vi "ConnectReseauDataManager.vi"(2 "entrée d'erreur":errorcluster) -> (0 "sortie d'erreur":errorcluster, 1 "Existe?":bool)   [LabVIEW 2017]
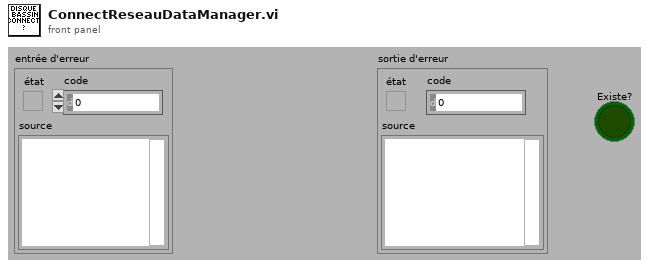
[diagram p1: front panel]
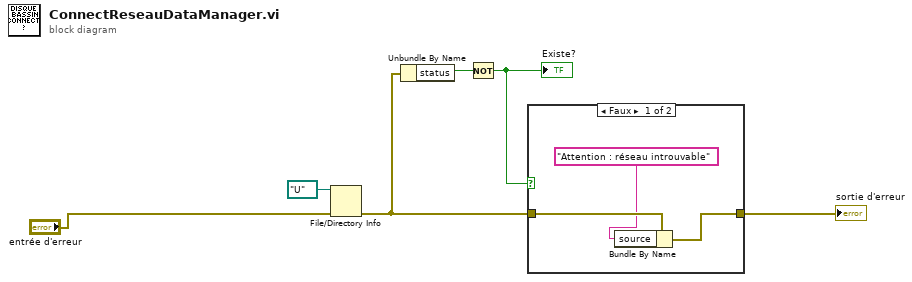
[diagram p0: block diagram]
diagram:
  n1 = File/Directory Info(path=path "U:/" ("chemin"), error in="entrée d'erreur") -> (error out=w4:errorcluster)  [unwired: 6 out]
  n2 = Unbundle By Name(w4) -> ("status"=w5:bool)
  n3 = Not(x=w5) -> (.not. x?=w6:bool)
  "Existe?" <- w6
  n4 = case shown="Faux" w6 {
    tunnel: w4 -> [w9 w10]
    tunnel: [w7 w10] -> w3
    frame False {
      n5 = Bundle By Name(cluster=w9, "source"="Attention : réseau introuvable") -> (w7:errorcluster)
    }
    frame True {
    }
  }
  "sortie d'erreur" <- w3
